vi "Read Type.vi"(11 "_Rename in":refnum<class "_Rename.lvclass">) -> (2 "Type":T1)   [LabVIEW 2025, in "_Rename.lvlib" / "_Rename.lvclass"]
uses:
  _Rename.lvclass
  _Rename.lvclass/_Rename.ctl
  _Shared/Type.ctl
  _Shared/_Shared.lvlib
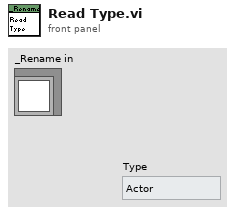
[diagram p1: front panel]
types:
  T1 = typedef "_Shared.lvlib/Type.ctl" = enum16{"Actor", "Msg"}
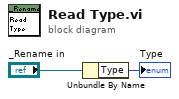
[diagram p0: block diagram]
diagram:
  n1 = Unbundle By Name("_Rename in") -> ("Type"=→"Type":T1)
